vi "AIDI-Start Tasks.vi"(0 "AO Tasks":T1[](array[typedef]), 7 "DO Tasks":T2, 11 "error in (no error)":errorcluster) -> (15 "error out":errorcluster)   [LabVIEW 2020]
uses:
  Typedefs/AIDI-DI Tasks.ctl
  Typedefs/AIDI-Task Specification.ctl
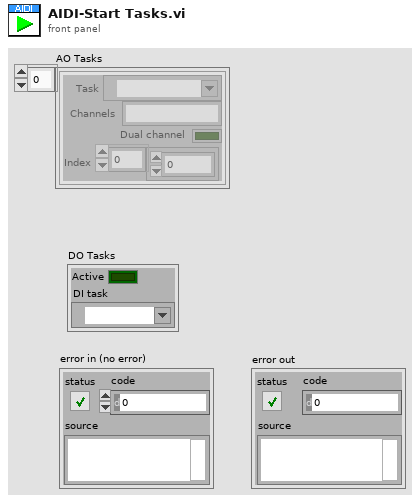
[diagram p1: front panel]
types:
  T1 = typedef "AIDI-Task Specification.ctl" = cluster{"Task":refnum<k21>, "Channels":string, "Dual channel":bool, "Index":i32[]}
  T2 = typedef "AIDI-DI Tasks.ctl" = cluster{"Active":bool, "DI task":refnum<k21>}
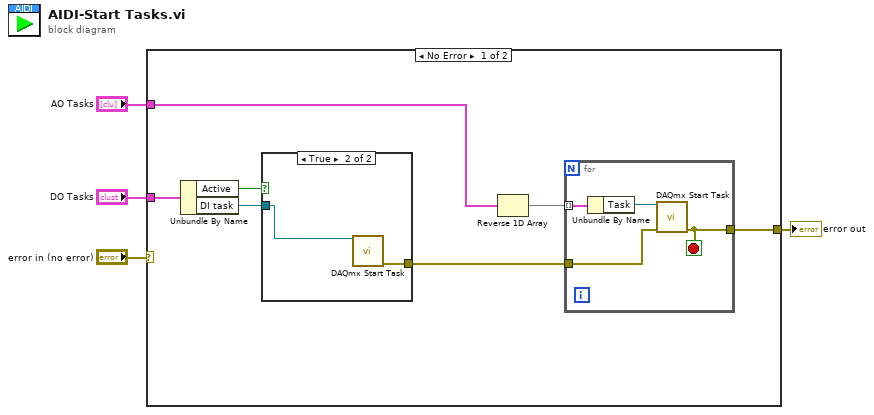
[diagram p0: block diagram]
diagram:
  n1 = case shown="No Error" "error in (no error)" {
    selector: "error in (no error)" -> [_ w18]
    tunnel: "DO Tasks" -> [w10 _]
    tunnel: [w5 w18] -> w3
    tunnel: "AO Tasks" -> [w8 _]
    frame No Error {
      n2 = Unbundle By Name(w10) -> ("Active"=w6:bool, "DI task"=w7:refnum<k21>)
      n3 = case shown="True" w6 {
        tunnel: w7 -> [_ w13]
        tunnel: [_ w12] -> w11
        frame False {
        }
        frame True {
          n4 = call <vilib>:"DAQmx Start Task.vi"("task/channels in"=w13) -> ("error out"=w12:errorcluster)  [unwired: 13 in, 1 out]
        }
      }
      n5 = Reverse 1D Array(array=w8) -> (reversed array=w9:T1[])
      n6 = for {
        tunnel: w9 -> [w17] mode=indexing
        tunnel: [w15] -> w5
        tunnel: w11 -> [w14]
        stop <- w15 stop-if-true
        n7 = Unbundle By Name(w17) -> ("Task"=w16:refnum<k21>)
        n8 = call <vilib>:"DAQmx Start Task.vi"("task/channels in"=w16, "error in"=w14) -> ("error out"=w15:errorcluster)  [unwired: 12 in, 1 out]
      }
    }
    frame Error {
    }
  }
  "error out" <- w3
